vi "Read_Plot_4ch.vi"() -> ()   [LabVIEW 2022 SP3]
uses:
  <vilib>/express/express analysis/Spectral/Block/exnSpectralBlock spectral measurements peak poly.vi
  <vilib>/express/express analysis/Spectral/Block/exnSpectralBlock spectral measurements peak DDT.vi
  <vilib>/express/express analysis/Spectral/XNode/ExpressSpectralMeasurementsBlockNode.xnode
panel:
  out "CH 0":dynamicdata(graph)
  out "CH 2":dynamicdata(graph)
  out "CH 1":dynamicdata(graph)
  out "CH 3":dynamicdata(graph)
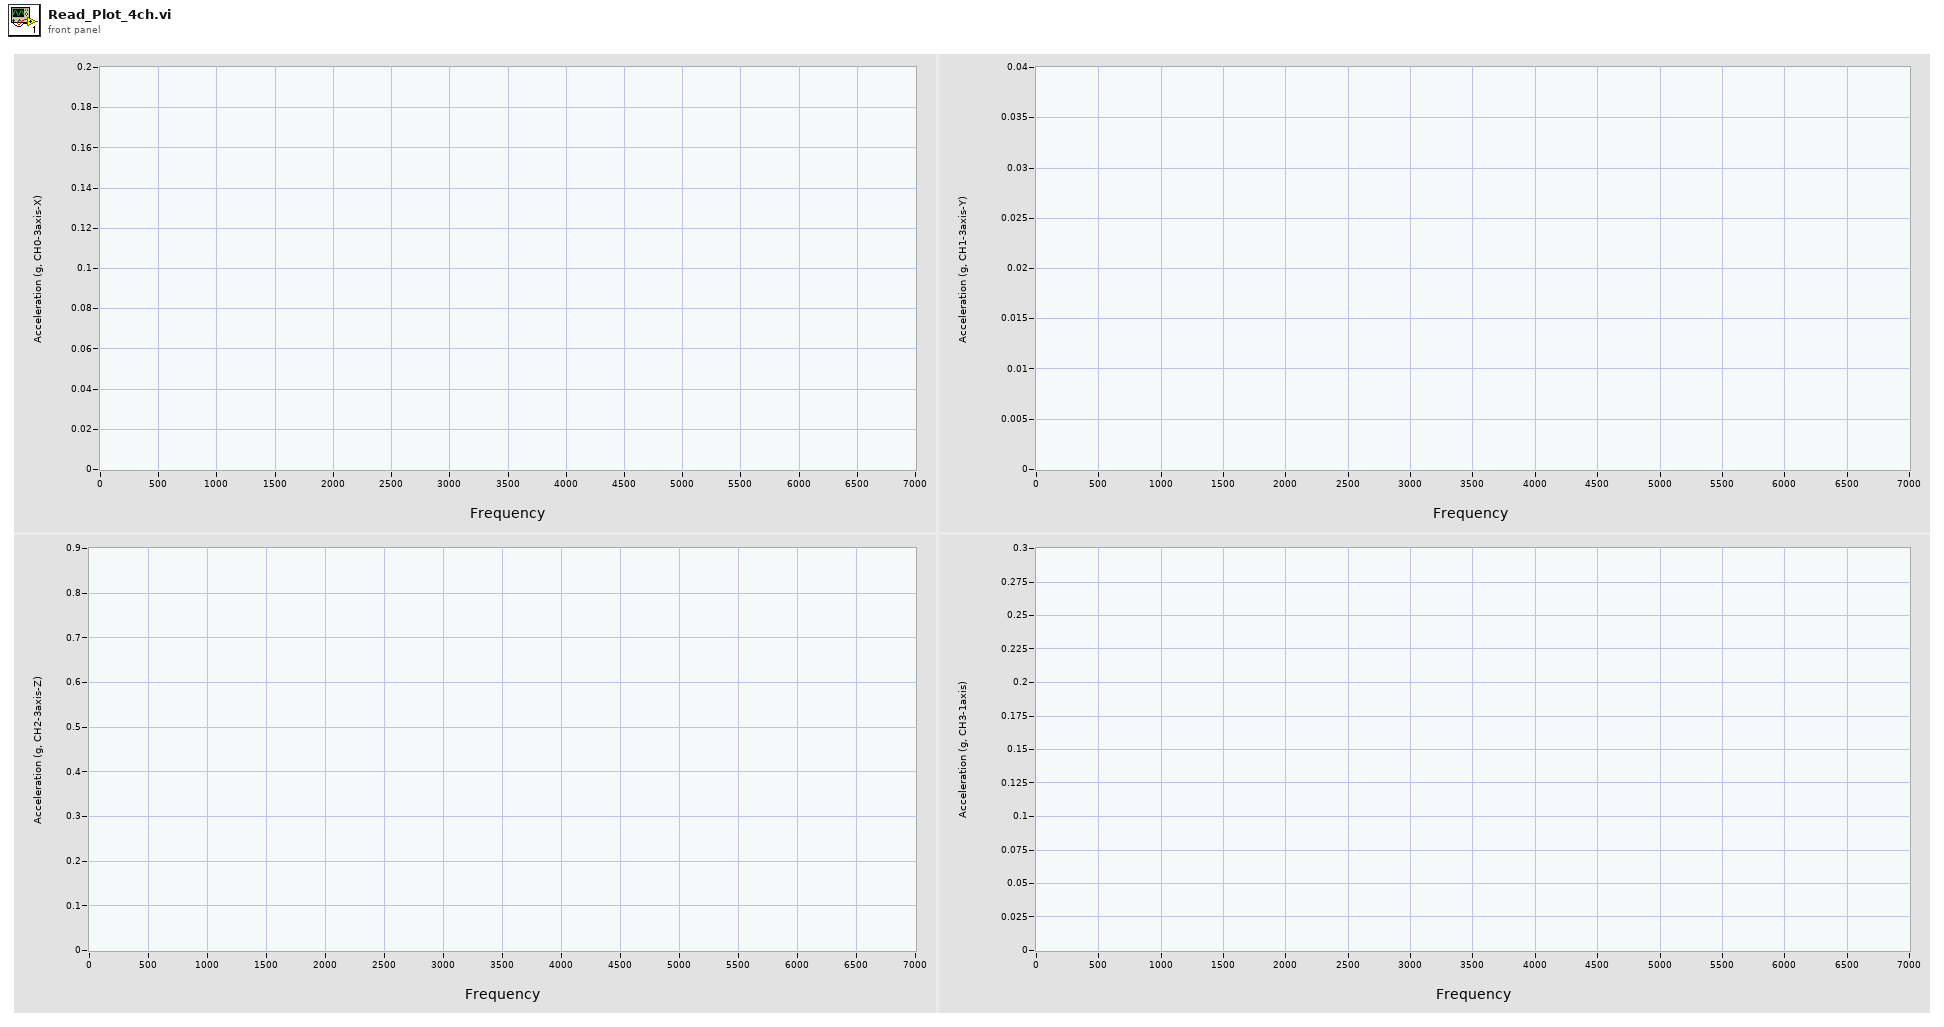
[diagram p1: front panel]
types:
  T1 = cluster{"averaging mode":u16, "weighting mode":u16, "number of averages":u32}
  T2 = cluster{"dB On (F)":bool, "unwrap phase (F)":bool, "convert to degree (F)":bool}
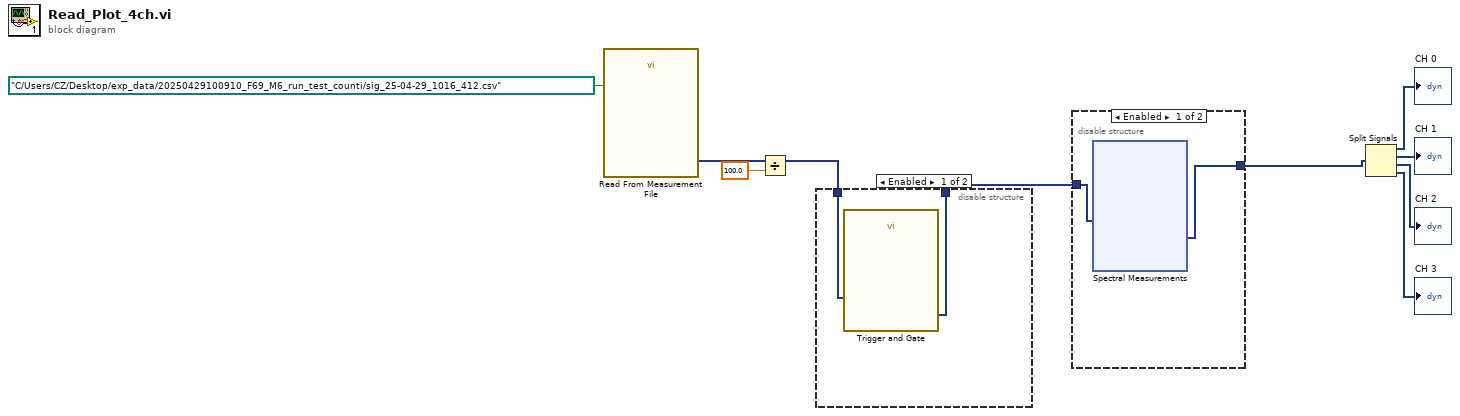
[diagram p0: block diagram]
diagram:
  n1 = call "Read From Measurement File"("Filename"=path "C:/Users/CZ/Desktop/exp_data/20250429100910_F69_M6_run_test_counti/sig_25-04-29_1016_412.csv") -> ("Signals"=w10:dynamicdata)  [unwired: 5 in, 5 out]
  n2 = Divide(x=w10, y=100.0) -> (x/y=w4:dynamicdata)
  n3 = disable-structure shown="Enabled" {
    disable-tunnel: w4 -> [w12 w13]
    disable-tunnel: [w11 w13] -> w3
    frame Enabled {
      n4 = call "Trigger and Gate"("Signals"=w12) -> ("Triggered Signals"=w11:dynamicdata)  [unwired: 7 in, 3 out]
    }
    frame Disabled {
    }
  }
  n5 = disable-structure shown="Enabled" {
    disable-tunnel: w3 -> [w15 w26]
    disable-tunnel: [w14 w26] -> w2
    frame Enabled {
      n6 = xnode "Spectral Measurements"("Signals"=w15) -> ("FFT - (Peak)"=w14:dynamicdata)  [unwired: 1 in, 2 out]
    }
    frame Disabled {
    }
  }
  n7 = Split Signals(w2) -> (→"CH 0":dynamicdata, →"CH 1":dynamicdata, →"CH 2":dynamicdata, →"CH 3":dynamicdata)  [unwired: 4 in]
